vi "json Insert String - string path.vi"(8 "error in (no error)":errorcluster, 9 "anything":string, 10 "path":string, 11 "JSON Document in":refnum<class "JSON Document.lvclass">) -> (0 "error out":errorcluster, 3 "JSON Document out":refnum<class "JSON Document.lvclass">)   [LabVIEW 2015, in "JSON Document.lvclass"]
uses:
  JSON Document.lvclass
  JSON Document.lvclass/JSON Document.ctl
  rapidjson wrapper/rapidjson wrapper.lvlib
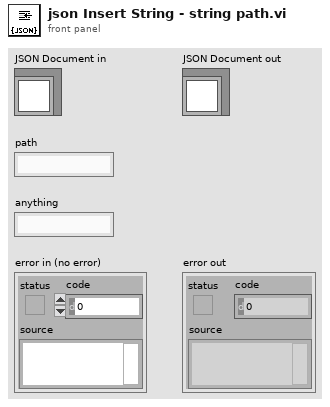
[diagram p1: front panel]
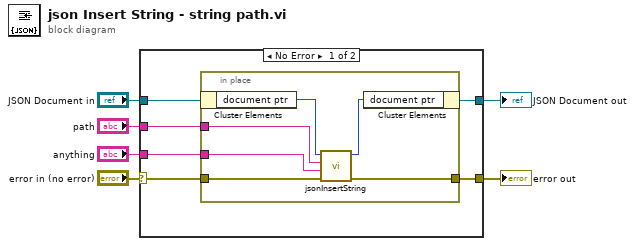
[diagram p0: block diagram]
diagram:
  n1 = case shown="No Error" "error in (no error)" {
    selector: "error in (no error)" -> [w8 w20]
    tunnel: [w9 w20] -> w5
    tunnel: [w11 w19] -> w3
    tunnel: "JSON Document in" -> [w12 w19]
    tunnel: "anything" -> [w7 _]
    tunnel: "path" -> [w10 _]
    frame No Error {
      n2 = in-place {
        in-place-border: w10 -> [w16]
        in-place-border: w8 -> [w15]
        in-place-border: [w14] -> w9
        in-place-border: w7 -> [w13]
        n3 = in-place-cluster #1(w12) -> ("document ptr"=w18:i64)
        n4 = call "jsonInsertString.vi"("error in (no error)"=w15, "value"=w13, "path"=w16, "d in"=w18) -> ("error out"=w14:errorcluster, "d out"=w17:i64)  [unwired: 6 in]
        n5 = in-place-cluster #1("document ptr"=w17) -> (w11:refnum<class "JSON Document.lvclass">)
      }
    }
    frame Error {
    }
  }
  "error out" <- w5
  "JSON Document out" <- w3
